vi "Select_Graph(SubVI).vi"(1 "PreviousArray":dbl[](array[numeric]), 2 "Finish Pos":i32, 3 "Start Pos":i32, 4 "InputArray":dbl[](array[numeric])) -> (0 "Output Graph":dbl[][](array[numeric]))   [LabVIEW 2014]
panel:
  # "СубВИ предназначено для отображения на графическом индикаторе\nзоны, которую выбрал оператор другим цветом"
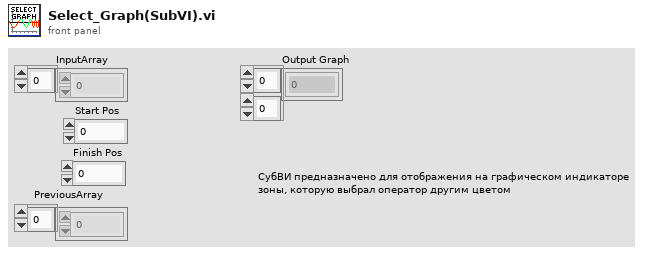
[diagram p1: front panel]
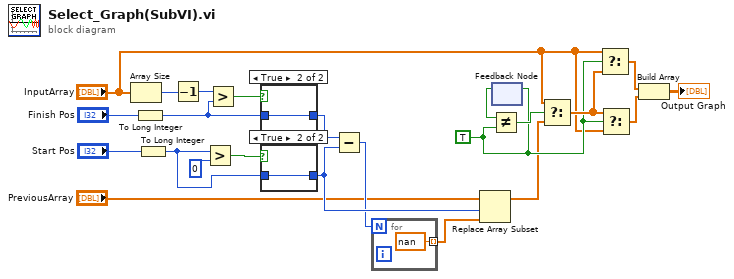
[diagram p0: block diagram]
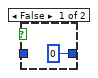
[diagram p2: hidden frame]
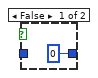
[diagram p3: hidden frame]
diagram:
  w5 = TRUE
  n1 = Array Size(array="InputArray") -> (size(s)=w23:i32)
  n2 = To Long Integer(number="Finish Pos") -> (32bit integer=w16:i32)
  n3 = To Long Integer(number="Start Pos") -> (32bit integer=w15:i32)
  n4 = Decrement(x=w23) -> (x-1=w22:i32)
  n5 = Greater?(x=w15, y=0) -> (0:w18:bool)
  n6 = Greater?(x=w22, y=w16) -> (0:w17:bool)
  n7 = case shown="True" w17 {
    tunnel: w16 -> [_ w25]
    tunnel: [0 w25] -> w14
    frame False {
    }
    frame True {
    }
  }
  n8 = case shown="True" w18 {
    tunnel: w15 -> [_ w27]
    tunnel: [0 w27] -> w13
    frame False {
    }
    frame True {
    }
  }
  n9 = Subtract(x=w14, y=w13) -> (x-y=w11:i32)
  n10 = for {
    N: w11 -> [_]
    tunnel: [nan ("t")] -> w12 mode=indexing
  }
  n11 = Replace Array Subset(array="PreviousArray", new element=w12, index=w13) -> (w4:dbl[])
  n12 = feedback #1() -> (w8:bool)  [unwired: 1 in]
  n13 = Not Equal?(x=w8, y=w5) -> (x != y?=w7:bool)
  n14 = feedback-in #1(w5) -> ()
  n15 = Select(t="InputArray", s=w7, f=w4) -> (s? t:f=w6:dbl[])
  n16 = Select(t="InputArray", s=w5, f=w6) -> (s? t:f=w9:dbl[])
  n17 = Select(t=w6, s=w5, f="InputArray") -> (s? t:f=w10:dbl[])
  n18 = Build Array(w9, w10) -> (→"Output Graph":dbl[][])
